vi "Read LogData.vi"(8 "error in (no error)":errorcluster, 11 "Log in":refnum<class "Log.lvclass">) -> (0 "error out":errorcluster, 2 "Log Data":T1, 3 "Log out":refnum<class "Log.lvclass">)   [LabVIEW 2017, in "Report_lib.lvlib" / "Log.lvclass"]
uses:
  Log.lvclass
  Log Data.ctl
  Log.lvclass/Log.ctl
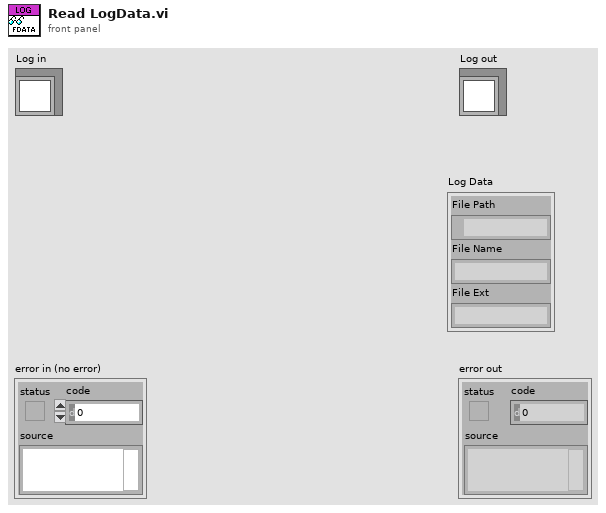
[diagram p1: front panel]
types:
  T1 = typedef "Log Data.ctl" = cluster{"File Path":path, "File Name":string, "File Ext":string}
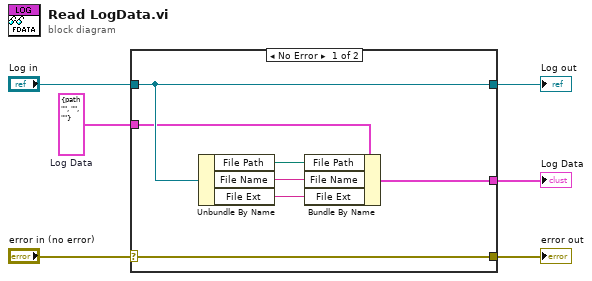
[diagram p0: block diagram]
diagram:
  w2 = T1 {"File Path"=path "", "File Name"="", "File Ext"=""}  # Log Data
  n1 = case shown="No Error" "error in (no error)" {
    selector: "error in (no error)" -> [w13 w15]
    tunnel: [w13 w15] -> w5
    tunnel: [w8 w16] -> w3
    tunnel: "Log in" -> [w8 w16]
    tunnel: w2 -> [w7 w14]
    tunnel: [w9 w14] -> w1
    frame No Error {
      n2 = Unbundle By Name(w8) -> ("File Path"=w12:path, "File Name"=w11:string, "File Ext"=w10:string)
      n3 = Bundle By Name(cluster=w7, "File Path"=w12, "File Name"=w11, "File Ext"=w10) -> (w9:T1)
    }
    frame Error {
    }
  }
  "error out" <- w5
  "Log out" <- w3
  "Log Data" <- w1
